vi "Test_ports_IO_xor_performance.vi"() -> ()   [LabVIEW 2018]
uses:
  <userlib>/_OpenG.lib/numeric/numeric.llb/Random Number Within Range - DBL__ogtk.vi
  Tracker.lvlib
  Libraries/TTL IO/TTL IO.lvlib
panel:
  out "Calculation is completed":bool
  out "Functions output is similar (within tested range)":bool
  in  "Old or New XOR function":bool
  out "OFF config":u32[](array[numeric])
  out "ON config":u32[](array[numeric])
  out "us per iteration":dbl
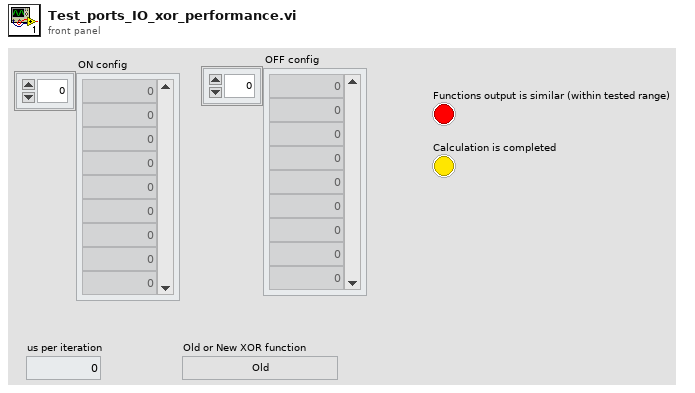
[diagram p1: front panel]
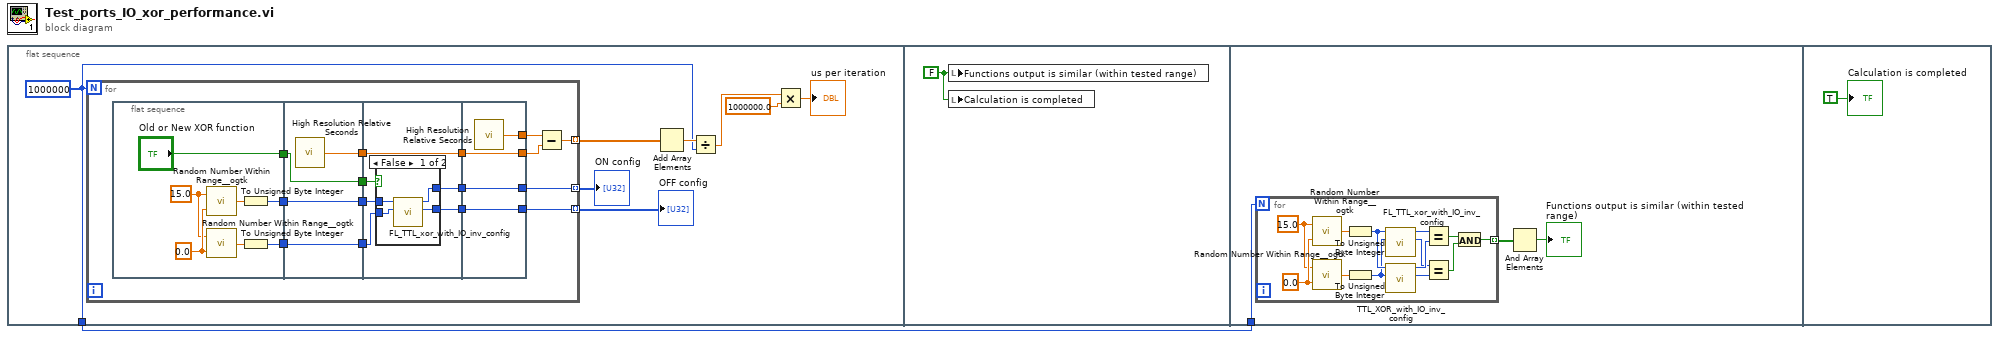
[diagram p0: block diagram]
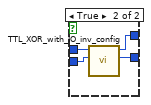
[diagram p2: hidden frame]
diagram:
  n1 = flat-sequence {
    tunnel: [w2] -> w1
    tunnel: w1 -> [w55]
    frame #0 {
      w2 = 1000000
      n2 = for {
        N: w2 -> [_]
        tunnel: [w20] -> w9 mode=indexing
        tunnel: [w15] -> w4 mode=indexing
        tunnel: [w13] -> w3 mode=indexing
        n3 = flat-sequence {
          tunnel: [w27] -> w19
          tunnel: [w26] -> w17
          tunnel: ["Old or New XOR function"] -> w10
          tunnel: [w35] -> w21
          tunnel: w19 -> [w34]
          tunnel: [w34] -> w18
          tunnel: w17 -> [w33]
          tunnel: [w33] -> w16
          tunnel: [w32] -> w11
          tunnel: w10 -> [w32]
          tunnel: [w41] -> w22
          tunnel: w21 -> [w41]
          tunnel: w18 -> [w40]
          tunnel: w16 -> [w39]
          tunnel: [w38] -> w14
          tunnel: [w37] -> w12
          tunnel: w11 -> [w36]
          tunnel: [w53] -> w24
          tunnel: [w52] -> w23
          tunnel: w22 -> [w52]
          tunnel: [w51] -> w15
          tunnel: w14 -> [w51]
          tunnel: [w50] -> w13
          tunnel: w12 -> [w50]
          frame #0 {
            w30 = 15.0 ("High")
            w31 = 0.0 ("High")
            n4 = call-poly <userlib>:"Random Number Within Range__ogtk.vi"("High"=w30, "Low"=w31) -> ("Random Number"=w29:dbl)  [unwired: 3 in]
            n5 = call-poly <userlib>:"Random Number Within Range__ogtk.vi"("High"=w30, "Low"=w31) -> ("Random Number"=w28:dbl)  [unwired: 3 in]
            n6 = To Unsigned Byte Integer(number=w29) -> (unsigned 8bit integer=w27:u8)
            n7 = To Unsigned Byte Integer(number=w28) -> (unsigned 8bit integer=w26:u8)
          }
          frame #1 {
            n8 = call <vilib>:"High Resolution Relative Seconds.vi"() -> ("relative seconds"=w35:dbl)
          }
          frame #2 {
            n9 = case shown="False" w36 {
              tunnel: w40 -> [w45 w49]
              tunnel: w39 -> [w44 w48]
              tunnel: [w43 w47] -> w38
              tunnel: [w42 w46] -> w37
              frame False {
                n10 = call "FL_TTL_xor_with_IO_inv_config.vi"("IO inversion config."=w44, "TTL port(s) config to fire"=w45) -> ("OFF config."=w42:u32, "ON config."=w43:u32)  [unwired: 8 in]
              }
              frame True {
                n11 = call "TTL_XOR_with_IO_inv_config.vi"("IO inversion config."=w48, "TTL port(s) config to fire"=w49) -> ("OFF config."=w46:u32, "ON config."=w47:u32)  [unwired: 8 in]
              }
            }
          }
          frame #3 {
            n12 = call <vilib>:"High Resolution Relative Seconds.vi"() -> ("relative seconds"=w53:dbl)
          }
        }
        n13 = Subtract(x=w24, y=w23) -> (x-y=w20:dbl)
      }
      "ON config" <- w4
      "OFF config" <- w3
      n14 = Add Array Elements(numeric array=w9) -> (sum=w8:dbl)
      n15 = Divide(x=w8, y=w2) -> (x/y=w7:dbl)
      n16 = Multiply(x=w7, y=1000000.0) -> (x*y=→"us per iteration":dbl)
    }
    frame #1 {
      w54 = FALSE ("Functions output is similar (within tested range)")
      n17 = local write "Functions output is similar (within tested range)"(w54) -> ()
      n18 = local write "Calculation is completed"(w54) -> ()
    }
    frame #2 {
      n19 = for {
        N: w55 -> [_]
        tunnel: [w58] -> w56 mode=indexing
        w69 = 15.0 ("High")
        w70 = 0.0 ("High")
        n20 = call-poly <userlib>:"Random Number Within Range__ogtk.vi"("High"=w69, "Low"=w70) -> ("Random Number"=w68:dbl)  [unwired: 3 in]
        n21 = call-poly <userlib>:"Random Number Within Range__ogtk.vi"("High"=w69, "Low"=w70) -> ("Random Number"=w67:dbl)  [unwired: 3 in]
        n22 = To Unsigned Byte Integer(number=w68) -> (unsigned 8bit integer=w66:u8)
        n23 = To Unsigned Byte Integer(number=w67) -> (unsigned 8bit integer=w65:u8)
        n24 = call "FL_TTL_xor_with_IO_inv_config.vi"("IO inversion config."=w65, "TTL port(s) config to fire"=w66) -> ("OFF config."=w62:u32, "ON config."=w64:u32)  [unwired: 8 in]
        n25 = call "TTL_XOR_with_IO_inv_config.vi"("IO inversion config."=w65, "TTL port(s) config to fire"=w66) -> ("OFF config."=w61:u32, "ON config."=w63:u32)  [unwired: 8 in]
        n26 = Equal?(x=w64, y=w63) -> (x = y?=w60:bool)
        n27 = Equal?(x=w62, y=w61) -> (x = y?=w59:bool)
        n28 = And(x=w60, y=w59) -> (x .and. y?=w58:bool)
      }
      n29 = And Array Elements(Boolean array=w56) -> (logical AND=→"Functions output is similar (within tested range)":bool)
    }
    frame #3 {
      "Calculation is completed" <- TRUE ("Calculation is completed")
    }
  }
